vi "DAC Configure FP View.vi"(8 "error in":errorcluster, 11 "DAC TC Temperature in":refnum<class "DAC TC Temp CryoSep.lvclass">) -> (0 "error out":errorcluster, 3 "DAC TC Temperature out":refnum<class "DAC TC Temp CryoSep.lvclass">)   [LabVIEW 2019, in "DAC.lvlib" / "DAC TC Temp CryoSep.lvclass"]
uses:
  DAC TC Temp CryoSep.lvclass
  Results/Results Method.ctl
  Results/Results.lvlib
  DAC.lvclass
  Results/Cryo Sep Results/Cryo Sep Results.lvclass
  C:/Users/krio/Documents/LV_Projects/test-stand/App/DAC/DAC.lvclass
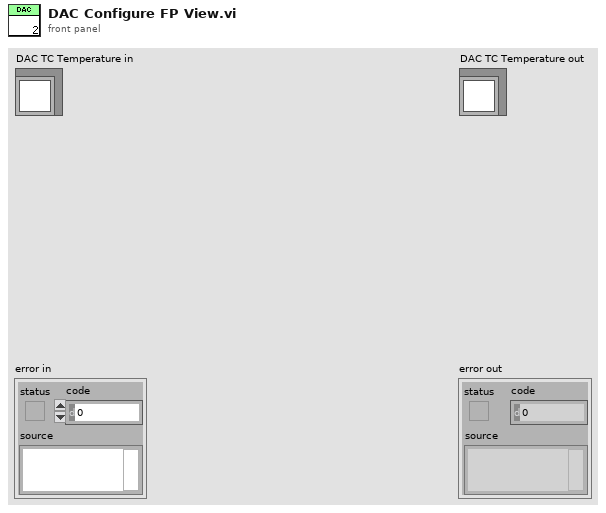
[diagram p1: front panel]
types:
  T1 = typedef "Results.lvlib/Results Method.ctl" = enum16{"Get", "Set"}
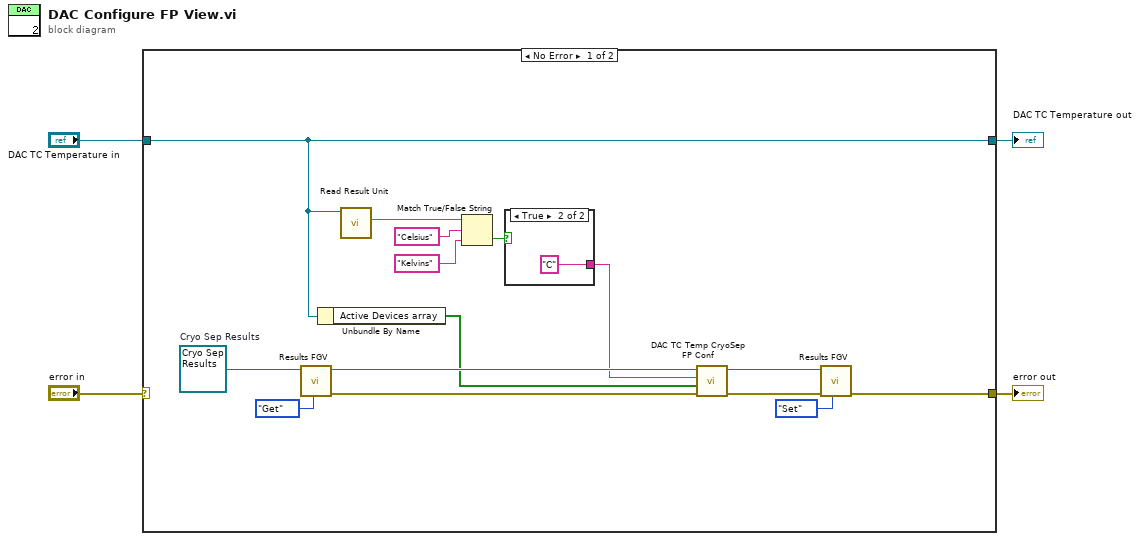
[diagram p0: block diagram]
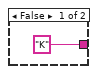
[diagram p2: hidden frame]
diagram:
  n1 = case shown="No Error" "error in" {
    selector: "error in" -> [_ w23]
    tunnel: [w19 w23] -> w1
    tunnel: [w16 w22] -> w2
    tunnel: "DAC TC Temperature in" -> [w16 w22]
    frame No Error {
      w11 = refnum<class "Cryo Sep Results.lvclass"> refnum  # Cryo Sep Results
      n2 = call-dynamic "Results FGV.vi"("Method"=Results_Method."Get", "Results in"=w11) -> ("error out"=w8:errorcluster, "Results out"=w10:refnum<class "Cryo Sep Results.lvclass">)  [unwired: 8 in]
      n3 = Unbundle By Name(w16) -> ("Active Devices array"=w7:bool[])
      n4 = call "Read Result Unit.vi"("DAC in"=w16) -> ("Unit"=w12:string)  [unwired: 8 in, 2 out]
      n5 = Match True/False String(2:"Kelvins" ("false string"), 3:"Celsius" ("true string"), 4:w12) -> (0:w13:bool)  [unwired: 1 out]
      n6 = case shown="True" w13 {
        tunnel: ["K" ("false string") "C" ("true string")] -> w6
        frame False {
        }
        frame True {
        }
      }
      n7 = call "DAC TC Temp CryoSep FP Conf.vi"("error in (no error)"=w8, "Used TC Temps"=w7, "Result Unit"=w6, "Cryo Sep Results in"=w10) -> ("error out"=w5:errorcluster, "Cryo Sep Results out"=w9:refnum<class "Cryo Sep Results.lvclass">)  [unwired: 6 in]
      n8 = call-dynamic "Results FGV.vi"("Method"=Results_Method."Set", "error in"=w5, "Results in"=w9) -> ("error out"=w19:errorcluster)  [unwired: 7 in, 1 out]
    }
    frame Error {
    }
  }
  "error out" <- w1
  "DAC TC Temperature out" <- w2
